vi "Periodic Tasks.vi"(8 "error in":errorcluster) -> ()   [LabVIEW 2016]
doc: "This VI runs in parallel to other tasks. It can contain as many user-defined periodic loops as you need. These can carry out PID or other sorts of timed response."
uses:
  <vilib>/Rock Robotics/WPI/Utilities/WPI_GetSetVariantRefNum.vi
  <vilib>/Rock Robotics/Network Tables/NT Write Numeric Array.vi
  Robot Global Data.vi
panel:
  out "AR Flutter":dbl
  out "Ang Flutter":dbl
  out "Ang Error":dbl
  out "Ang Min":dbl
  out "AR Min":dbl
  out "AR Error":dbl
  out "Ang Max":dbl
  out "AR Max":dbl
  out "Z Error":dbl
  out "Y Error":dbl
  out "X Error":dbl
  out "X Flutter":dbl
  out "Y Flutter":dbl
  out "Z Flutter":dbl
  out "X Min":dbl
  out "Y Min":dbl
  out "Z Min":dbl
  out "X Max":dbl
  out "Y Max":dbl
  out "Z Max":dbl
  in  "stop":bool
  out "X Acceleration":dbl
  out "Y Acceleration":dbl
  out "Z Acceleration":dbl
  out "X Accel 2":dbl(graph)
  out "Y Accel 2":dbl(graph)
  out "Z Accel 2":dbl(graph)
  out "X Flut 2":dbl(graph)
  out "Y Flut 2":dbl(graph)
  out "Z Flut 2":dbl(graph)
  out "Connected":bool
  out "Connection Count":i32
  out "Remainder Angle":dbl
  out "Angular Rate 2":dbl
  out "Angle 2":dbl
  in  "error in 2":errorcluster
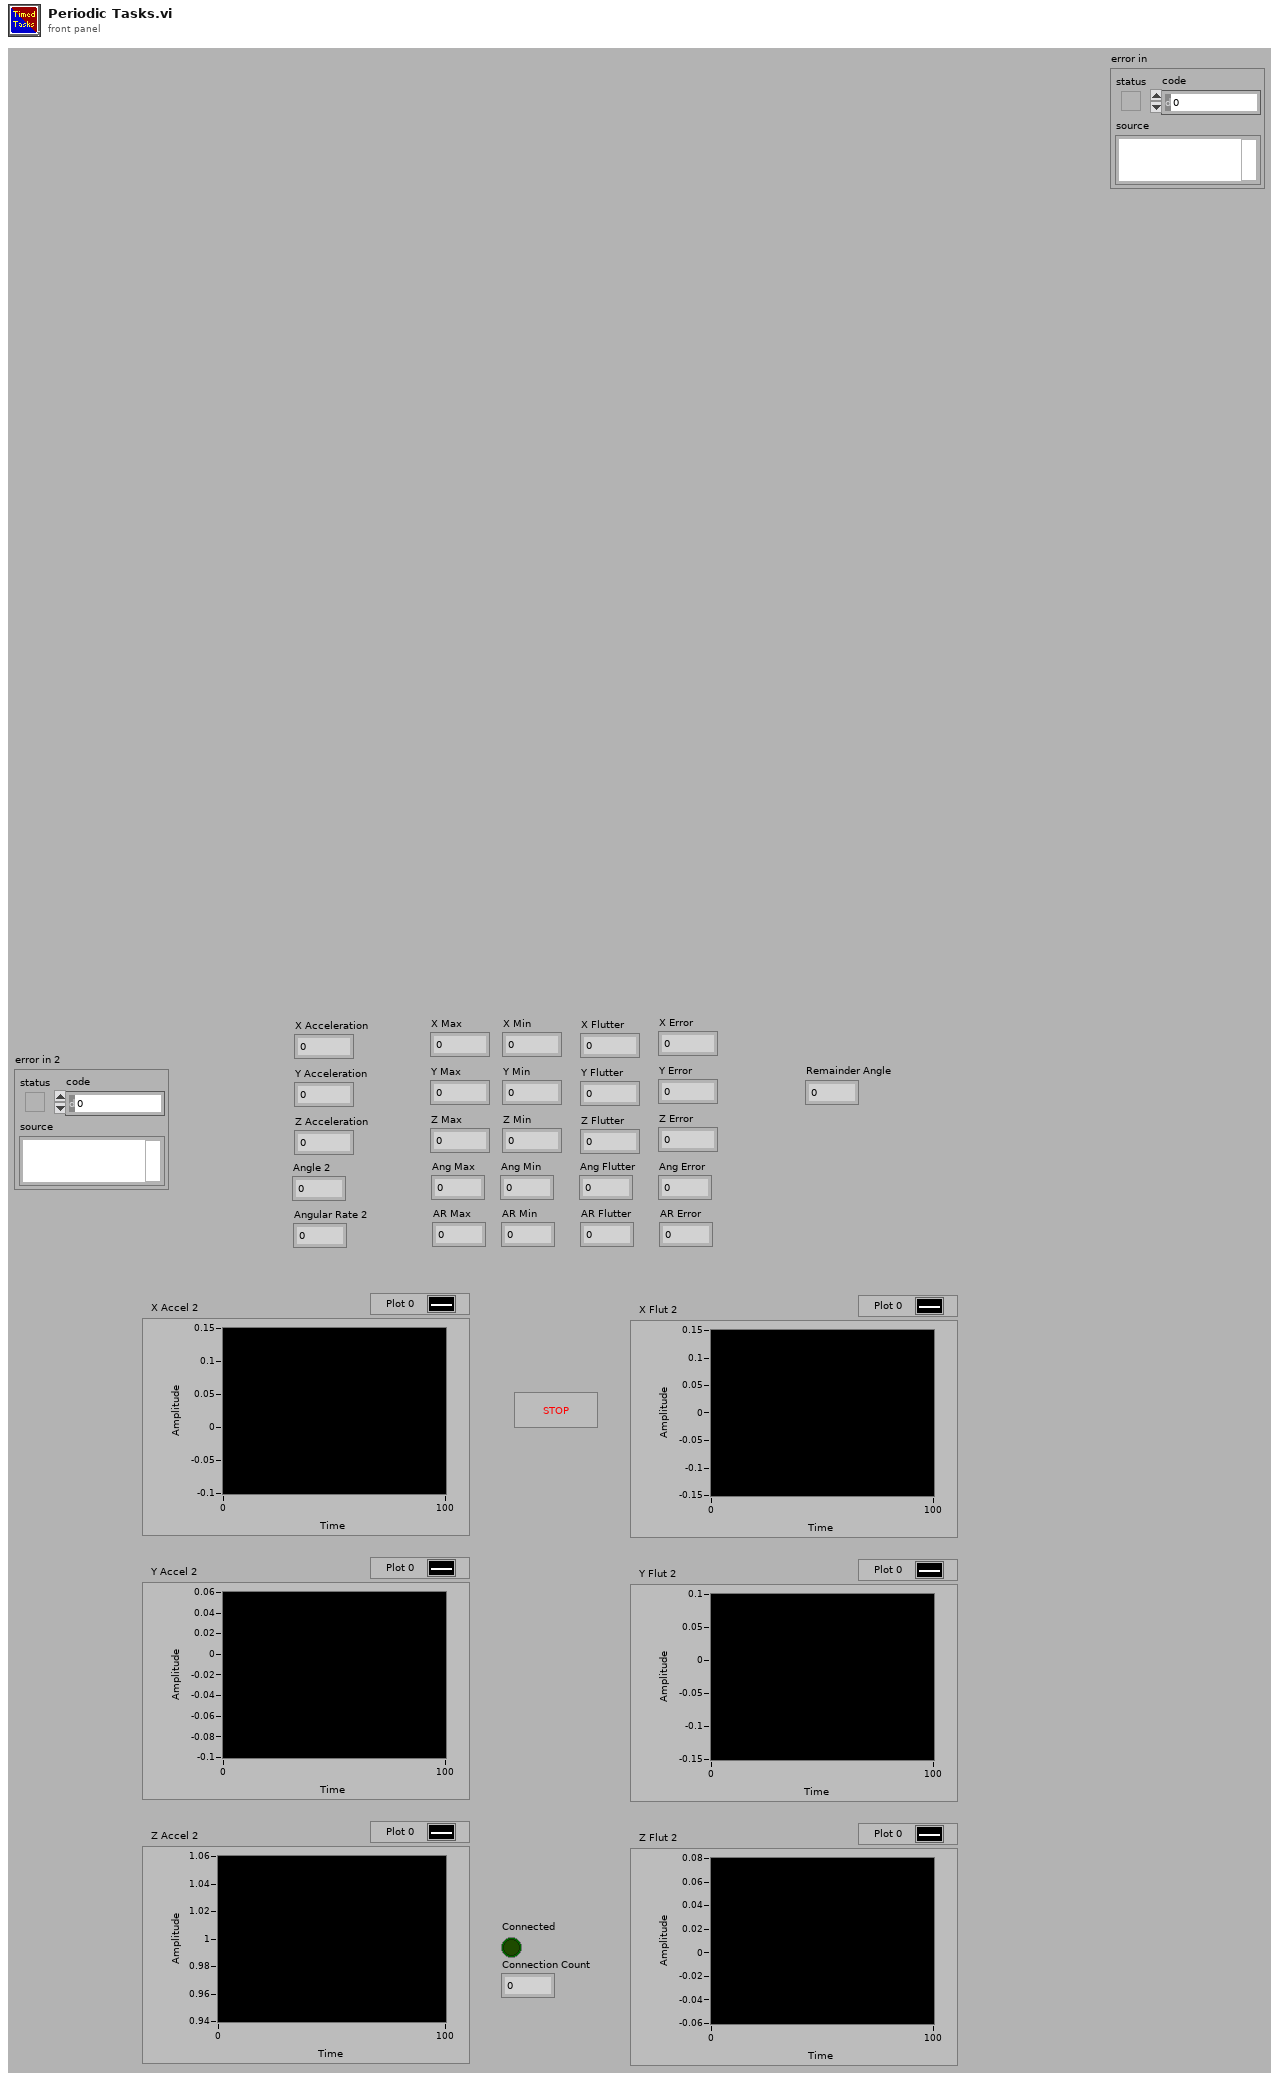
[diagram p1: front panel]
types:
  T1 = typedef "WPI_GyroDevRef.ctl" = cluster{"DevStatus":errorcluster, "Analog Channel":T2, "Offset":dbl, "Gain (VoltsPerDegree/Second)":dbl, "Gyro Type":enum16{"Analog", "XRS450"}, "Handle":i32, "SPI Bus":T3, "Device Found":bool, "Sample Rate":dbl, "Calibrate On Open":bool}
  T2 = typedef "FPGA_AIChannel.ctl" = enum8{"AI 0", "AI 1", "AI 2", "AI 3", "AI MXP 0", "AI MXP 1", "AI MXP 2", "AI MXP 3", "Invalid"}
  T3 = typedef "spi_bus.ctl" = enum16{"SPI On-Board, CS0", "SPI On-Board, CS1", "SPI On-Board, CS2", "SPI On-Board, CS3", "SPI MXP", "Invalid"}
  T4 = typedef "WPI_AccelerometerDevRef.ctl" = cluster{"DevStatus":errorcluster, "Scaling":T5, "Analog Channels":T6, "I2C Bus":T7, "SPI Bus":T3, "Accel Range":T8, "ADXL Axes":T9, "Handle":i32, "Device Address":u8, "Accel Type":enum16{"Analog", "ADXL345 I2C", "ADXL345 SPI", "Internal", "ADXL362 SPI"}}
  T5 = typedef "WPI_AccelerometerScaling.ctl" = cluster{"Gain (VoltsPerG)":dbl, "Center Voltage":dbl}
  T6 = typedef "WPI_AccelerometerAnalogChannels.ctl" = cluster{"X-Axis":T2, "Y-Axis":T2, "Z-Axis":T2}
  T7 = typedef "i2c_bus.ctl" = enum16{"I2C On-Board", "I2C MXP", "Invalid"}
  T8 = typedef "ADXL345 Range.ctl" = u8
  T9 = typedef "WPI_AccelerometerADXL345 Axes.ctl" = cluster{"X-Axis":bool, "Y-Axis":bool, "Z-Axis":bool}
  T10 = typedef "WPI_JoystickDevRef.ctl" = cluster{"Device":T11}
  T11 = typedef "WPI_JoystickDeviceEnum.ctl" = enum16{"USB 0", "USB 1", "USB 2", "USB 3", "USB 4", "USB 5"}
  T12 = typedef "WPI_RobotDriveDevRef.ctl" = cluster{"DevStatus":errorcluster, "Motors[]":T13[], "Square Inputs":bool, "Max Output":dbl}
  T13 = typedef "WPI_MotorControlDeviceRef.ctl" = cluster{"DeviceStatus":errorcluster, "Type":T14, "PWM":cluster{"PWM Channel":T15, "DeadBand":T16}, "CAN":cluster{"Device Number":u8, "SetOutput VI Ref":variant, "GetOutput VI Ref":variant, "Enable VI Ref":variant, "Disable VI Ref":variant, "Data":variant}, "Invert":bool}
  T14 = typedef "WPI_MotorControlType.ctl" = enum16{"PWM", "CAN"}
  T15 = typedef "FPGA_DIOPWMChannel.ctl" = enum8{"PWM 0", "PWM 1", "PWM 2", "PWM 3", "PWM 4", "PWM 5", "PWM 6", "PWM 7", "PWM 8", "PWM 9", "PWM MXP 0", "PWM MXP 1", "PWM MXP 2", "PWM MXP 3", "PWM MXP 4", "PWM MXP 5", "PWM MXP 6", "PWM MXP 7", "PWM MXP 8", "PWM MXP 9", "Invalid"}
  T16 = typedef "WPI_PWMDeadband.ctl" = cluster{"Name":string, "maxPositivePwm":i32, "minPositivePwm":i32, "centerPwm":i32, "maxNegativePwm":i32, "minNegativePwm":i32, "angularRange":u16}
  T17 = cluster{"X-Axis":dbl, "Y-Axis":dbl, "Z-Axis":dbl}
  T18 = cluster{"JoystickDevRef":T10, "RobotDriveDevRef":T12}
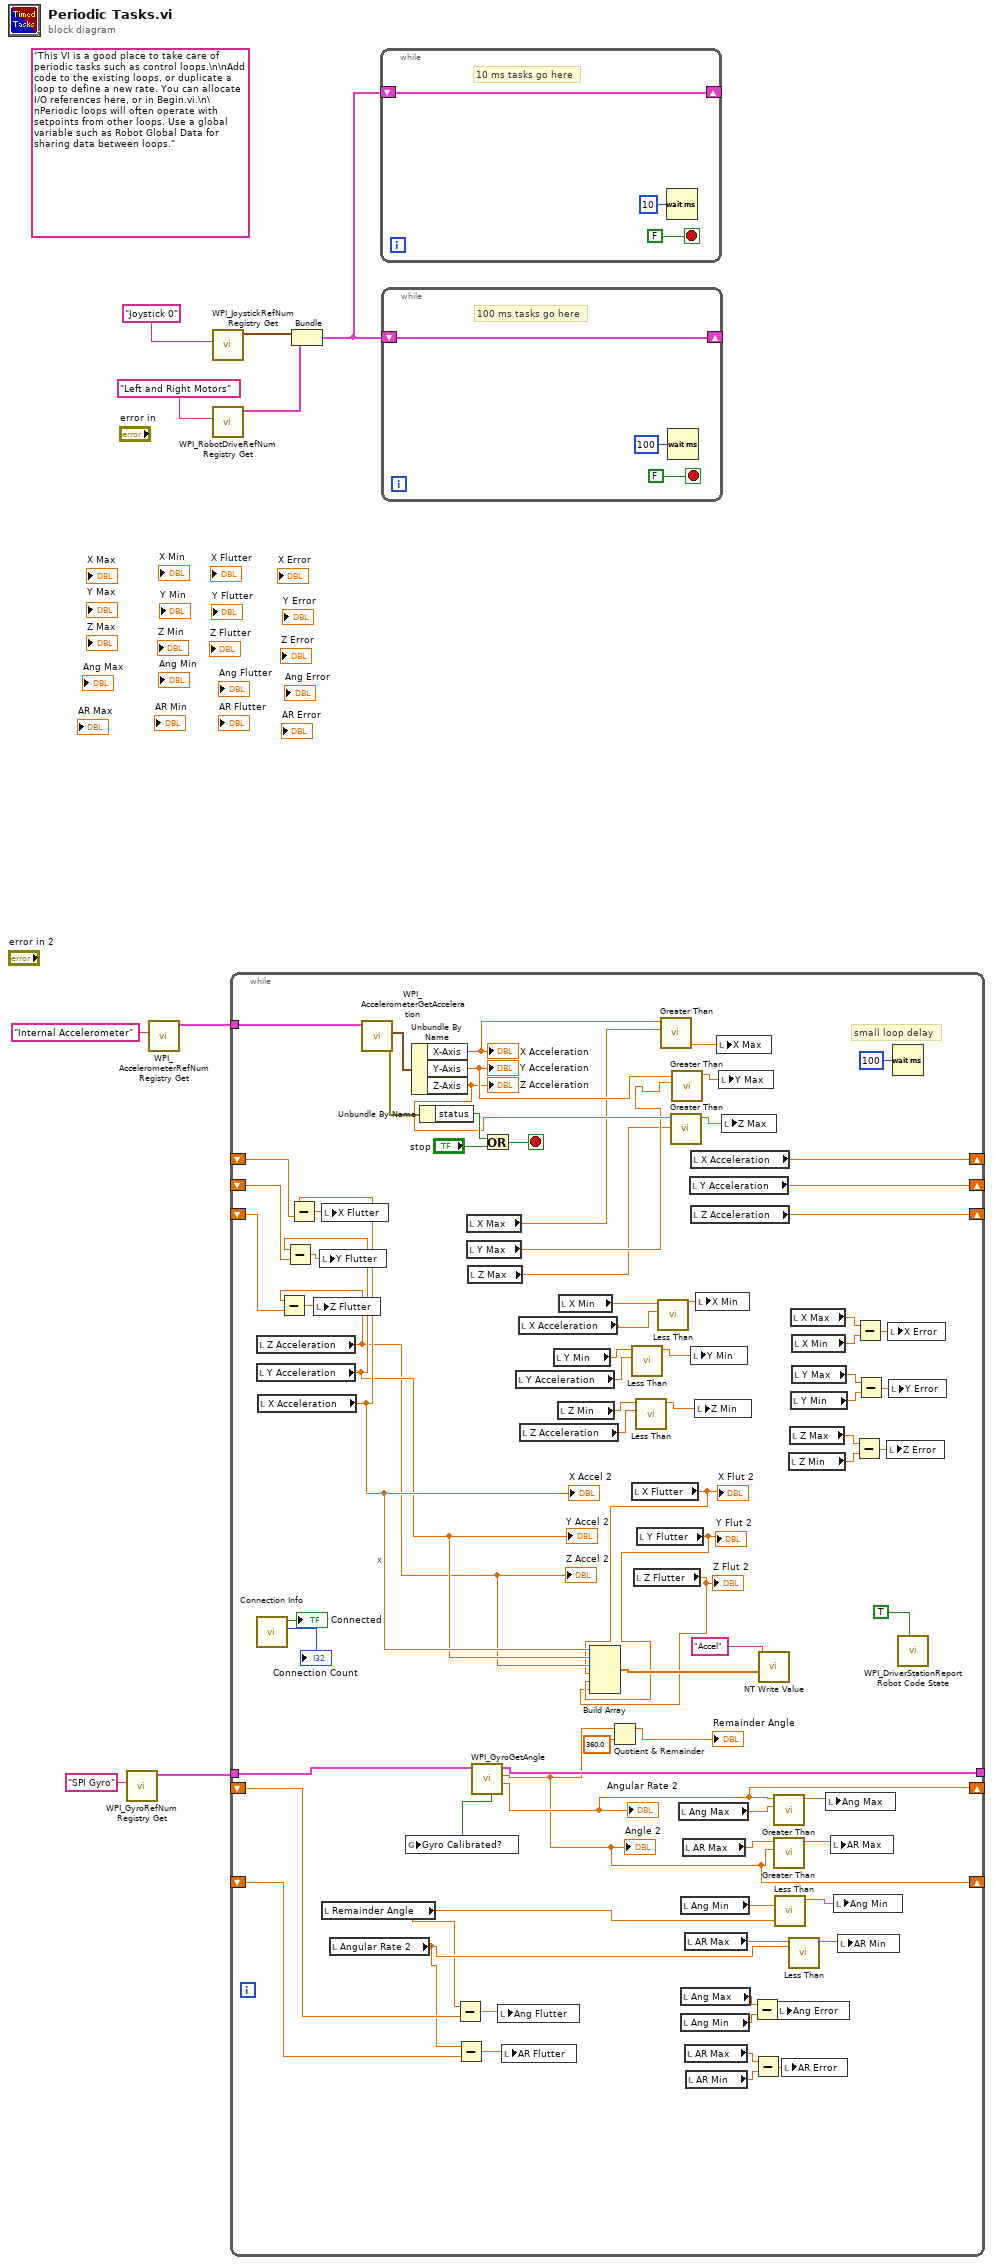
[diagram p0: block diagram]
diagram:
  (unwired) "This VI is a good place to take care of periodic tasks such as control loops.\n\nAdd code to the existing loops, or duplicate a loop to define a new rate. You can allocate I/O references here, or in Begin.vi.\n\nPeriodic loops will often operate with setpoints from other loops. Use a global variable such as Robot Global Data for sharing data between loops."
  n1 = call <vilib>:"WPI_GyroRefNum Registry Get.vi"("refnum name"="SPI Gyro") -> ("GyroDevRef"=w1:T1)  [unwired: 9 in, 1 out]
  n2 = call <vilib>:"WPI_AccelerometerRefNum Registry Get.vi"("refnum name"="Internal Accelerometer") -> ("AccelerometerDevRef"=w2:T4)  [unwired: 9 in, 1 out]
  n3 = call <vilib>:"WPI_JoystickRefNum Registry Get.vi"("refnum name"="Joystick 0") -> ("JoystickDevRef"=w7:T10)  [unwired: 1 in, 9 out]
  n4 = call <vilib>:"WPI_RobotDriveRefNum Registry Get.vi"("refnum name"="Left and Right Motors") -> ("RobotDriveDevRef"=w6:T12)  [unwired: 1 in, 9 out]
  n5 = while {
    shift-right: [w72] -> _
    shift-left: _ -> [w67]
    shift-right: [w71] -> _
    shift-left: _ -> [w68]
    shift-right: [w70] -> _
    shift-left: _ -> [w69]
    tunnel: w1 -> [w21]
    tunnel: [w43] -> _
    shift-right: [w37] -> _
    shift-left: _ -> [w32]
    shift-right: [w12] -> _
    shift-left: _ -> [w29]
    tunnel: w2 -> [w22]
    stop <- w86 stop-if-true
    # "X"
    # "small loop delay"
    n6 = local read "Z Acceleration"() -> (w48:dbl)
    "Z Accel 2" <- w48
    n7 = local read "Y Acceleration"() -> (w49:dbl)
    "Y Accel 2" <- w49
    n8 = call <vilib>:"Connection Info.vi"() -> ("Connection Count"=→"Connection Count":i32, "Connected"=→"Connected":bool)  [unwired: 10 in]
    n9 = local read "X Acceleration"() -> (w50:dbl)
    "X Accel 2" <- w50
    n10 = Subtract(x=w48, y=w69) -> (x-y=w64:dbl)
    n11 = Subtract(x=w49, y=w68) -> (x-y=w65:dbl)
    n12 = Subtract(x=w50, y=w67) -> (x-y=w66:dbl)
    n13 = local write "Z Flutter"(w64) -> ()
    n14 = local write "Y Flutter"(w65) -> ()
    n15 = local write "X Flutter"(w66) -> ()
    n16 = local read "Remainder Angle"() -> (w10:dbl)
    n17 = local read "Angular Rate 2"() -> (w11:dbl)
    n18 = call <vilib>:"WPI_AccelerometerGetAcceleration.vi"("AccelerometerDevRef"=w22) -> ("error out"=w85:errorcluster, "Accelerations"=w87:T17)  [unwired: 8 in, 1 out]
    n19 = Unbundle By Name(w87) -> ("X-Axis"=w84:dbl, "Y-Axis"=w82:dbl, "Z-Axis"=w80:dbl)
    "X Acceleration" <- w84
    "Y Acceleration" <- w82
    "Z Acceleration" <- w80
    n20 = Unbundle By Name(w85) -> ("status"=w90:bool)
    n21 = Subtract(x=w10, y=w32) -> (x-y=w31:dbl)
    n22 = Subtract(x=w11, y=w29) -> (x-y=w30:dbl)
    n23 = local read "X Max"() -> (w19:dbl)
    n24 = local read "Y Max"() -> (w18:dbl)
    n25 = local read "Z Max"() -> (w17:dbl)
    n26 = call <vilib>:"WPI_GyroGetAngle.vi"("GyroDevRef"=w21) -> ("Angular Rate"=w37:dbl, "Angle"=w12:dbl, "GyroDevRef"=w43:T1, "Calibrated?"=w20:bool)  [unwired: 6 in, 1 out]
    "Angular Rate 2" <- w37
    "Angle 2" <- w12
    n27 = global write "Robot Global Data.vi" "Gyro Calibrated?"(w20) -> ()
    n28 = Or(x=w90, y="stop") -> (x .or. y?=w86:bool)
    n29 = local write "Ang Flutter"(w31) -> ()
    n30 = local write "AR Flutter"(w30) -> ()
    n31 = local read "Y Acceleration"() -> (w15:dbl)
    n32 = local read "X Acceleration"() -> (w16:dbl)
    n33 = local read "Z Acceleration"() -> (w14:dbl)
    n34 = local read "Y Min"() -> (w76:dbl)
    n35 = local read "Z Min"() -> (w73:dbl)
    n36 = local read "X Min"() -> (w77:dbl)
    n37 = Quotient & Remainder(x=w12, y=360.0) -> (x-y*floor(x/y)=→"Remainder Angle":dbl)  [unwired: 1 out]
    n38 = call "Less Than.vi"("Numeric 3"=w15, "Numeric in"=w76) -> ("Numeric out"=w75:dbl)  [unwired: 9 in]
    n39 = local read "X Flutter"() -> (w46:dbl)
    "X Flut 2" <- w46
    n40 = local read "Z Flutter"() -> (w44:dbl)
    "Z Flut 2" <- w44
    n41 = call "Less Than.vi"("Numeric 3"=w14, "Numeric in"=w73) -> ("Numeric out"=w74:dbl)  [unwired: 9 in]
    n42 = local read "Y Flutter"() -> (w45:dbl)
    "Y Flut 2" <- w45
    n43 = Build Array(w50, w49, w48, w46, w45, w44) -> (w47:dbl[])
    n44 = call "Less Than.vi"("Numeric 3"=w16, "Numeric in"=w77) -> ("Numeric out"=w78:dbl)  [unwired: 9 in]
    n45 = call "Greater Than.vi"("Numeric 5"=w19, "Numeric 6"=w84) -> ("Numeric 7"=w83:dbl)  [unwired: 9 in]
    n46 = call "Greater Than.vi"("Numeric 5"=w17, "Numeric 6"=w80) -> ("Numeric 7"=w79:dbl)  [unwired: 9 in]
    n47 = call "Greater Than.vi"("Numeric 5"=w18, "Numeric 6"=w82) -> ("Numeric 7"=w81:dbl)  [unwired: 9 in]
    n48 = local read "Ang Max"() -> (w13:dbl)
    n49 = local read "Ang Min"() -> (w36:dbl)
    n50 = local read "Ang Max"() -> (w23:dbl)
    n51 = local read "Ang Min"() -> (w24:dbl)
    n52 = local read "AR Max"() -> (w39:dbl)
    n53 = local read "AR Max"() -> (w34:dbl)
    n54 = local read "AR Max"() -> (w28:dbl)
    n55 = local read "AR Min"() -> (w27:dbl)
    n56 = local read "Y Acceleration"() -> (w71:dbl)
    n57 = local read "X Acceleration"() -> (w72:dbl)
    n58 = local read "Z Acceleration"() -> (w70:dbl)
    n59 = local write "Y Min"(w75) -> ()
    n60 = local write "Z Min"(w74) -> ()
    n61 = local write "X Min"(w78) -> ()
    n62 = local write "X Max"(w83) -> ()
    n63 = local write "Y Max"(w81) -> ()
    n64 = local write "Z Max"(w79) -> ()
    n65 = Subtract(x=w23, y=w24) -> (x-y=w25:dbl)
    n66 = Subtract(x=w28, y=w27) -> (x-y=w26:dbl)
    n67 = call-poly <vilib>:"NT Write Value.vi"("Numeric Array"=w47, "Name"="Accel") -> ()  [unwired: 9 in, 1 out]
    n68 = call "Greater Than.vi"("Numeric 5"=w13, "Numeric 6"=w37) -> ("Numeric 7"=w40:dbl)  [unwired: 9 in]
    n69 = call "Greater Than.vi"("Numeric 5"=w12, "Numeric 6"=w39) -> ("Numeric 7"=w38:dbl)  [unwired: 9 in]
    n70 = call "Less Than.vi"("Numeric 3"=w10, "Numeric in"=w36) -> ("Numeric out"=w35:dbl)  [unwired: 9 in]
    n71 = local write "Ang Error"(w25) -> ()
    n72 = local write "AR Error"(w26) -> ()
    n73 = local read "Z Min"() -> (w56:dbl)
    n74 = call "Less Than.vi"("Numeric 3"=w11, "Numeric in"=w34) -> ("Numeric out"=w33:dbl)  [unwired: 9 in]
    n75 = local read "Z Max"() -> (w57:dbl)
    n76 = local read "X Max"() -> (w63:dbl)
    n77 = local read "Y Min"() -> (w59:dbl)
    n78 = local read "X Min"() -> (w62:dbl)
    n79 = local read "Y Max"() -> (w58:dbl)
    n80 = local write "Ang Max"(w40) -> ()
    n81 = local write "AR Max"(w38) -> ()
    n82 = local write "Ang Min"(w35) -> ()
    n83 = local write "AR Min"(w33) -> ()
    n84 = Subtract(x=w57, y=w56) -> (x-y=w55:dbl)
    n85 = Subtract(x=w63, y=w62) -> (x-y=w61:dbl)
    n86 = Subtract(x=w58, y=w59) -> (x-y=w60:dbl)
    n87 = local write "Z Error"(w55) -> ()
    n88 = local write "X Error"(w61) -> ()
    n89 = local write "Y Error"(w60) -> ()
    n90 = Wait (ms)(milliseconds to wait=u32 100) -> ()  [unwired: 1 out]
    n91 = call <vilib>:"WPI_DriverStationReport Robot Code State.vi"("Test"=TRUE) -> ()  [unwired: 10 in, 1 out]
  }
  n92 = Bundle("JoystickDevRef"=w7, "RobotDriveDevRef"=w6) -> (w5:T18)  [unwired: 1 out]
  n93 = while {
    shift-right: [w91] -> _
    shift-left: w5 -> [w91]
    stop <- FALSE stop-if-true
    # "10 ms tasks go here"
    n94 = Wait (ms)(milliseconds to wait=u32 10) -> ()  [unwired: 1 out]
  }
  n95 = while {
    shift-right: [w94] -> _
    shift-left: w5 -> [w94]
    stop <- FALSE stop-if-true
    # "100 ms tasks go here"
    n96 = Wait (ms)(milliseconds to wait=u32 100) -> ()  [unwired: 1 out]
  }
